vi "Do.vi"(8 "error in (no error)":errorcluster, 10 "Message in":refnum<class "Stop Message.lvclass">, 11 "Execute":refnum<class "Execute.lvclass">) -> (0 "error out":errorcluster, 2 "Message out":refnum<class "Stop Message.lvclass">, 3 "Execute":refnum<class "Execute.lvclass">)   [LabVIEW 2018, in "QMH_Class.lvlib" / "TestManager.lvlib" / "Stop Message.lvclass"]
uses:
  Stop Message.lvclass
  Execute_class/Execute.lvclass
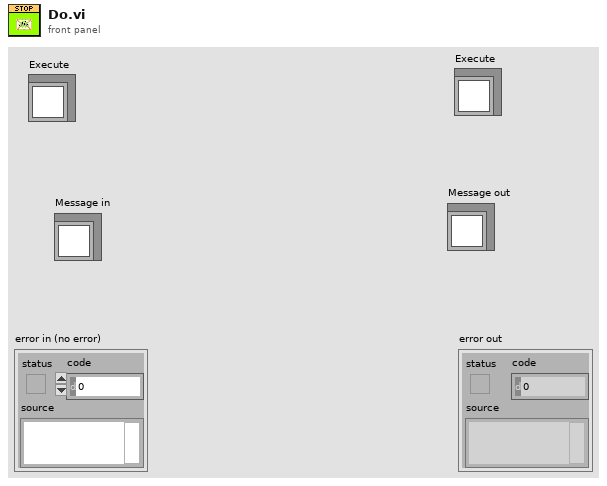
[diagram p1: front panel]
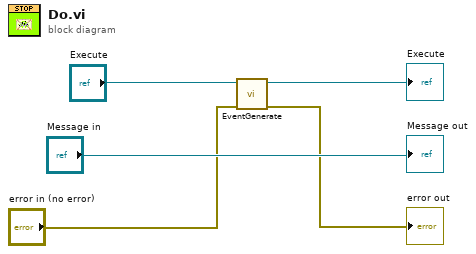
[diagram p0: block diagram]
diagram:
  n1 = call "EventGenerate.vi"("error in (no error)"="error in (no error)", "Execute"="Execute") -> ("error out"=→"error out":errorcluster, "Execute"=→"Execute":refnum<class "Execute.lvclass">)  [unwired: 8 in]
  "Message out" <- "Message in"
